vi "UHR-Fleezers Control (host) -TL FB Corrected Ronen semipassive - stepping.vi"(0 "Tab Control":T5(tab)=enum."Trap Control (RF)") -> ()   [LabVIEW 2013] (continued)
  n79 = xnode "Read/Write Control"("FPGA VI Reference In"=w138, "error in"=w158, "ai count"="AI Count (ticks)", "Interlace ON/OFF"=w124, "Number Interlace Cycles"=w123, "AI1 Sets to FIFO"=w251, "FB On/Off Set 1"=w250, "FB On/Off Set 2"=w249, "Interlace Off Parameters"=w122, "FB Setpoint Set 1"=w241, "FB Setpoint Set 2"=w240, "FB Gains Set 1"=w238, "FB Gains Set 2"=w237, "FB output range 1"=w140, "FB output range 2"=w140, "Cycles per step"=w222, "Scan BD"=w234, "Number of scans"=w218, "Scan steps"=w223, "Scan freq.  increment"=w224, "AO1"=w206, "AO2"=w205, "Scan freq.  increment (MCL)"=w199, "Scan steps (MCL)"=w198, "Cycles per step (MCL)"=w197, "Number of scans (MCL)"=w196, "MCL count"=w121, "Cont. Scan (MCL)"=w195, "MCL Scan Axis"=w189, "1D or 2D Scan?"=w141, "N of AI1 Int Acq Sets"=w179, "Freq or Amp switch first"="Freq or Amp switch first", "Freq switch delay"="Freq switch delay", "Amp switch delay"="Amp switch delay", "Swap F1 and F2"="Swap F1 and F2", "APD Acq Rate Count"=w146, "APD to FIFO"=FALSE, "APD Gate Operating Mode"="APD Gate", "APD Gate ON Count"="APD Gate ON Count", "APD Gate OFF Count"="APD Gate OFF Count", "Invert APD Gate"="Invert APD Gate", "DIO count 1 (ticks)"="DIO count 1 (ticks)", "DIO count 2 (ticks)"="DIO count 2 (ticks)", "DIO count 3 (ticks)"="DIO count 3 (ticks)", "APD 1 AO scale factor"="APD 1 AO Mult.", "APD 2 AO scale factor"="APD 2 AO Mult.", "Diff FB Measurement?"=w3, "Dynamic Force FB (Ronen)"=w2, "Negate Diff?"=w1) -> ("FPGA VI Reference Out"=w116:T20, "error out"=w118:errorcluster)  [unwired: 1 in]
  n80 = local read "Green Laser ON/Interlacing"() -> (w119:bool)
  n81 = local read "Green laser mode"() -> (w120:enum32{"Laser ON", "Laser OFF", "Interlace"})
  n82 = local read "GI Frequency, OFF count"() -> (w112:u32)
  n83 = local read "GI Frequency, ON count"() -> (w111:u32)
  n84 = Multiply(x="Current When FB OFF (%)", y=655.35) -> (x*y=w102:dbl)
  n85 = local read "Green FB Count"() -> (w110:u32)
  n86 = Multiply(x="Green FB Setpoint (mV)", y=3.2767) -> (x*y=w99:dbl)
  n87 = To Unsigned Word Integer(number=w102) -> (unsigned 16bit integer=w100:u16)
  n88 = local read "Invert GI"() -> (w114:bool)
  n89 = To Word Integer(number=w99) -> (16bit integer=w97:i16)
  n90 = case shown="True" w119 {
    tunnel: w120 -> [_ w271]
    tunnel: [enum32{"Laser ON", "Laser OFF", "Interlace"}."Laser OFF" ("Green laser mode") w271] -> w113
    frame False {
    }
    frame True {
    }
  }
  n91 = local read "Trap Pos. AI1 X Pre-scale"() -> (w68:u16)
  n92 = local read "Trap Pos FB Monitor\nT1 or T2"() -> (w75:bool)
  n93 = local read "Trap Pos FB Int Count"() -> (w63:u16)
  n94 = local read "Trap Pos FB Negate Action"() -> (w74:bool)
  n95 = local read "Trap Pos. FB Offset Factor"() -> (w73:i64)
  n96 = local read "Trap Pos. FB Mult Factor"() -> (w72:i64)
  n97 = local read "Trap Pos. FB Gains"() -> (w70:T11)
  n98 = local read "Trap Pos. FB Range"() -> (w71:T12)
  n99 = xnode "Read/Write Control"("FPGA VI Reference In"=w116, "error in"=w118, "Green interlace ON count 2"=w111, "Green interlace OFF count 2"=w112, "Invert GI 2"=w114, "Operating Mode 2"=w113, "Green FB Gains"="Green FB Gains", "Green FB Setpoint"=w97, "Green FB On/Off"="Green FB On/Off", "Current Out"=w100, "Green int current ON count adj"="Green int current ON count adj", "Green FB Count"=w110, "Operating Mode"=w113, "Green interlace OFF count"=w112, "Green interlace ON count"=w111, "Invert GI"=w114, "Trap Pos FB Monitor T1 or T2"=w75, "Trap Pos FB Negate Action"=w74, "Trap Pos. FB Offset Factor"=w73, "Trap Pos. FB Mult Factor"=w72, "Trap Pos. FB Range"=w71, "Trap Pos. FB Gains"=w70, "Force feedback"=FALSE, "AI1 X Scale"=w68, "Trap Pos to FIFO"=TRUE, "Trap Pos FB Int Count"=w63) -> ("FPGA VI Reference Out"=w115:T20, "error out"=w117:errorcluster)
  n100 = xnode "Invoke Method"("FPGA VI Reference In"=w115, "error in"=w117, "Requested Depth"="Trap AI FIFO Depth") -> ("FPGA VI Reference Out"=w78:T20, "error out"=w77:errorcluster)  [unwired: 1 out]
  n101 = xnode "Invoke Method"("FPGA VI Reference In"=w78, "error in"=w77, "Requested Depth"="Trap Position FIFO Depth") -> ("FPGA VI Reference Out"=w65:T20, "error out"=w64:errorcluster)  [unwired: 1 out]
  n102 = flat-sequence {
    tunnel: w139 -> [w276]
    tunnel: [w276] -> w138
    tunnel: [w275] -> w20
    tunnel: [w274] -> w137
    tunnel: [w272] -> w135
    tunnel: [w273] -> w136
    frame #0 {
      w273 = T17 {"Minimum"=60.0, "Maximum"=90.0, "Increment"=1.0} ("Min Max Inc")
      w272 = T17 {"Minimum"=0.0, "Maximum"=75.0, "Increment"=1.0} ("Data Entry Limits")
      w275 = T17 {"Minimum"=60.0, "Maximum"=90.0, "Increment"=1.0} ("Min Max Inc")
      w274 = T17 {"Minimum"=0.0, "Maximum"=75.0, "Increment"=1.0} ("Data Entry Limits")
      n103 = property on="BD 2 Frequency 1 (MHz)" class="DigNum (strict)"("Data Range"=w273) -> ()  [unwired: 2 in, 2 out]
      n104 = property on="BD 2 Frequency 3 (MHz)" class="DigNum (strict)"("Data Range"=w273) -> ()  [unwired: 2 in, 2 out]
      n105 = property on="BD 2 Frequency 2 (MHz)" class="DigNum (strict)"("Data Range"=w273) -> ()  [unwired: 2 in, 2 out]
      n106 = property on="BD 1 Frequency 1 (MHz)" class="DigNum (strict)"("Data Range"=w275) -> ()  [unwired: 2 in, 2 out]
      n107 = property on="BD 1 Frequency 2 (MHz)" class="DigNum (strict)"("Data Range"=w275) -> ()  [unwired: 2 in, 2 out]
      n108 = property on="BD 1 Frequency 3 (MHz)" class="DigNum (strict)"("Data Range"=w275) -> ()  [unwired: 2 in, 2 out]
      n109 = property on="BD 2 Amplitude 1 (%)" class="DigNum (strict)"("Data Range"=w272) -> ()  [unwired: 2 in, 2 out]
      n110 = property on="BD 2 Amplitude 2 (%)" class="DigNum (strict)"("Data Range"=w272) -> ()  [unwired: 2 in, 2 out]
      n111 = property on="BD 2 Amplitude 3 (%)" class="DigNum (strict)"("Data Range"=w272) -> ()  [unwired: 2 in, 2 out]
      n112 = property on="BD 1 Amplitude 3 (%)" class="DigNum (strict)"("Data Range"=w274) -> ()  [unwired: 2 in, 2 out]
      n113 = property on="BD 1 Amplitude 2 (%)" class="DigNum (strict)"("Data Range"=w274) -> ()  [unwired: 2 in, 2 out]
      n114 = property on="BD 1 Amplitude 1 (%)" class="DigNum (strict)"("Data Range"=w274) -> ()  [unwired: 2 in, 2 out]
      "X RF Frequency Limits (MHz)" <- w275
      "X RF Amplitude Limits (%)" <- w274
      "Y RF Amplitude Limits (%)" <- w272
      "Y RF Frequency Limits (MHz)" <- w273
    }
  }
  n115 = xnode "Invoke Method"("FPGA VI Reference In"=w65, "error in"=w64) -> ("FPGA VI Reference Out"=w42:T20, "error out"=w41:errorcluster)  [unwired: 1 in]
  n116 = flat-sequence "Initial FPGA Loop Relative Phase Adjustment" {
    tunnel: "Initial Phase Adjustment (APD 2 Gate)" -> [w278]
    tunnel: "Initial Phase Adjustment (GI) 2" -> [w279]
    tunnel: "Initial Phase Adj. (MCL)" -> [w280]
    tunnel: w41 -> [w281]
    tunnel: w42 -> [w282]
    tunnel: "Initial Phase Adjustment (GI)" -> [w283]
    tunnel: "Initial Phase Adjustment (AI1)" -> [w284]
    tunnel: [w284] -> w51
    tunnel: [w283] -> w50
    tunnel: [w282] -> w49
    tunnel: [w281] -> w48
    tunnel: [w280] -> w47
    tunnel: [w279] -> w46
    tunnel: [w278] -> w45
    tunnel: [w296] -> w164
    tunnel: [w290] -> w162
    tunnel: "Initial Phase Adjustment (APD Acq)" -> [w289]
    tunnel: "Initial Phase Adjustment (APD 1 Gate)" -> [w288]
    tunnel: "Initial Phase Adjustment (Green FB)" -> [w287]
    tunnel: w51 -> [w295]
    tunnel: w50 -> [w294]
    tunnel: w49 -> [w293]
    tunnel: w48 -> [w292]
    tunnel: w47 -> [w291]
    tunnel: w46 -> [w286]
    tunnel: w45 -> [w285]
    tunnel: w164 -> [w298]
    tunnel: [w299] -> w163
    tunnel: w162 -> [w299]
    tunnel: [w298] -> w161
    tunnel: w163 -> [w302]
    tunnel: w161 -> [w301]
    tunnel: [w304] -> w160
    tunnel: [w303] -> w159
    tunnel: [w306] -> w40
    tunnel: [w307] -> w43
    tunnel: w160 -> [w307]
    tunnel: w159 -> [w306]
    frame #0 {
      n117 = Wait (ms)(milliseconds to wait=u32 1000) -> ()  [unwired: 1 out]
    }
    frame #1 {
      n118 = xnode "Read/Write Control"("FPGA VI Reference In"=w293, "error in"=w292, "Phase count adjustment"=w295, "Phase count adjustment (GI)"=w294, "Phase count adjustment (MCL)"=w291, "Phase Count Adjustment (APD Acq)"=w289, "Phase count adjustment (APD 1 Gate)"=w288, "Phase count adjustment (APD 2 Gate)"=w285, "Phase count adjustment (Green FB)"=w287, "Phase count adjustment (GI) 2"=w286) -> ("FPGA VI Reference Out"=w290:T20, "error out"=w296:errorcluster)
    }
    frame #2 {
      n119 = Wait (ms)(milliseconds to wait=u32 1000) -> ()  [unwired: 1 out]
    }
    frame #3 {
      w300 = TRUE
      n120 = xnode "Read/Write Control"("FPGA VI Reference In"=w302, "error in"=w301, "+ phase"=w300, "+ phase (GI)"=w300, "+ phase (MCL)"=w300, "+ phase (APD Acq)"=w300, "+ phase (APD 1 Gate)"=w300, "+ phase (APD 2 Gate)"=w300, "+ phase (Green FB)"=w300, "+ phase (GI) 2"=w300) -> ("FPGA VI Reference Out"=w303:T20, "error out"=w304:errorcluster)
    }
    frame #4 {
      n121 = Wait (ms)(milliseconds to wait=u32 1000) -> ()  [unwired: 1 out]
    }
  }
  n122 = Unbundle By Name(w20) -> ("Minimum"=w19:dbl, "Maximum"=w18:dbl)
  n123 = local read "Phase adj. (Green FB)"() -> (w133:i16)
  n124 = local read "Phase adj. (GI) 2"() -> (w103:i16)
  n125 = local read "Phase adjust (MCL)"() -> (w190:i16)
  n126 = local read "Phase adj. (AI1)"() -> (w192:i16)
  n127 = local read "Phase adj. (GI)"() -> (w191:i16)
  n128 = Multiply(x=w19, y=w17) -> (x*y=w15:dbl)
  n129 = Multiply(x=w18, y=w17) -> (x*y=w16:dbl)
  n130 = Multiply(x=49152000.0, y=6.0) -> (x*y=w9:dbl)
  n131 = Scale By Power Of 2(n=w14, x=w15) -> (x*2^n=w11:dbl)
  n132 = Scale By Power Of 2(n=w14, x=w16) -> (x*2^n=w10:dbl)
  n133 = xnode "Read/Write Control"("FPGA VI Reference In"=w40, "error in"=w43, "Phase count adjustment"=w192, "Phase count adjustment (GI)"=w191, "Phase count adjustment (MCL)"=w190, "Phase Count Adjustment (APD Acq)"="Phase Adj. (APD Acq)", "Phase count adjustment (APD 1 Gate)"="Phase Adj. (APD 1 Gate)", "Phase count adjustment (APD 2 Gate)"="Phase Adj. (APD 2 Gate)", "Phase count adjustment (Green FB)"=w133, "Phase count adjustment (GI) 2"=w103) -> ("FPGA VI Reference Out"=w39:T20, "error out"=w38:errorcluster)
  n134 = Divide(x=w10, y=w9) -> (x/y=w7:dbl)
  n135 = Divide(x=w11, y=w9) -> (x/y=w8:dbl)
  n136 = To Unsigned Quad Integer(1:w8) -> (0:w5:u64)
  n137 = To Unsigned Quad Integer(1:w7) -> (0:w4:u64)
  n138 = call "Initialize RF boards - interlace 3.vi"("error in"=w38, "FPGA VI Reference In"=w39) -> ("FPGA VI Reference Out"=w6:T20)  [unwired: 1 out]
  n139 = xnode "Read/Write Control"("FPGA VI Reference In"=w6, "FB Min Frequency"=w5, "FB Max Frequency"=w4) -> ()  [unwired: 1 in, 2 out]
  n140 = call "set RF board frequency - interlace.vi"("Board 2 Frequency Limits"=w136, "Board 1 Frequency Limits"=w20, "FPGA VI Reference In"=w6, "Board 2 Frequency 3 (MHz)"="BD 2 Frequency 3 (MHz)", "Board 1 Frequency 3 (MHz)"="BD 1 Frequency 3 (MHz)", "Board 2 Frequency 2 (MHz)"="BD 2 Frequency 2 (MHz)", "Board 2 Frequency 1 (MHz)"="BD 2 Frequency 1 (MHz)", "Board 1 Frequency 2 (MHz)"="BD 1 Frequency 2 (MHz)", "Board 1 Frequency 1  (MHz)"="BD 1 Frequency 1 (MHz)") -> ("error out"=w262:errorcluster, "FPGA VI Reference Out"=w263:T20)  [unwired: 1 in]
  n141 = call "set RF board amplitude - interlace.vi"("Board 2 Amplitude Limits"=w135, "Board 1 Amplitude Limits"=w137, "error in"=w262, "FPGA VI Reference In"=w263, "Board 2 Amplitude 3 (%)"="BD 2 Amplitude 3 (%)", "Board 1 Amplitude 3 (%)"="BD 1 Amplitude 3 (%)", "Board 2 Amplitude 2 (%)"="BD 2 Amplitude 2 (%)", "Board 2 Amplitude 1 (%)"="BD 2 Amplitude 1 (%)", "Board 1 Amplitude 2 (%)"="BD 1 Amplitude 2 (%)", "Board 1 Amplitude 1 (%)"="BD 1 Amplitude 1 (%)") -> ("error out"=w36:errorcluster, "FPGA VI Reference Out"=w37:T20)
  n142 = flat-sequence {
    tunnel: w37 -> [w316]
    tunnel: w36 -> [w315]
    tunnel: [w314] -> w255
    tunnel: [w313] -> w254
    tunnel: [w320] -> w253
    tunnel: w255 -> [w320]
    tunnel: [w319] -> w252
    tunnel: w254 -> [w319]
    tunnel: w253 -> [w329]
    tunnel: w252 -> [w328]
    tunnel: [w327] -> w32
    tunnel: [w322] -> w31
    tunnel: [w332] -> w60
    tunnel: [w336] -> w44
    tunnel: w32 -> [w336]
    tunnel: w31 -> [w331]
    frame #0 {
      n143 = local read "Trap 1 (ON/OFF)"() -> (w308:bool)
      n144 = xnode "Read/Write Control"("FPGA VI Reference In"=w316, "error in"=w315, "Direct RF Box  Communication"=FALSE) -> ("FPGA VI Reference Out"=w314:T20, "error out"=w313:errorcluster)
      n145 = local write "Saving..."(FALSE ("Saving Data")) -> ()
      n146 = local write "Stop All"(FALSE ("Stop All")) -> ()
      n147 = local write "Index"(1.0 ("Index")) -> ()
      n148 = property on="Trap 1 ON" class="Bool (strict)"("Value"=w308) -> ()  [unwired: 2 in, 2 out]
      "Manipulating Trap" <- FALSE ("Manipulating Trap")
    }
    frame #1 {
      n149 = local read "Trap 2 (ON/OFF)"() -> (w318:bool)
      n150 = Wait (ms)(milliseconds to wait=u32 50) -> ()  [unwired: 1 out]
      n151 = property on="Trap 2 ON" class="Bool (strict)"("Val(Sgnl)"=w318) -> ()  [unwired: 2 in, 2 out]
    }
    frame #2 {
      n152 = local read "Scan Range (nm)"() -> (w323:dbl)
      n153 = xnode "Read/Write Control"("FPGA VI Reference In"=w329, "error in"=w328, "FPGA Controls  RF Box"=TRUE ("Direct RF Box  Communication")) -> ("FPGA VI Reference Out"=w327:T20, "error out"=w322:errorcluster)
      n154 = call "Update messages.vi"("Message to add"="UHR-Fleezers ready.", "Old message string"="") -> ("New message string"=w326:string)
      n155 = local write "Messages"(w326) -> ()
      n156 = property on="Scan Range (nm)" class="DigNum (strict)"("Val(Sgnl)"=w323) -> ()  [unwired: 2 in, 2 out]
    }
    frame #3 {
      n157 = call "hamilton_controller.vi"("error in"=w331, "action"=T21."CONNECT") -> ("error out"=w333:errorcluster)  [unwired: 9 in]
      n158 = call "hamilton_controller.vi"("error in"=w333, "action"=T21."INITIALIZE VALVES") -> ("error out"=w332:errorcluster)  [unwired: 9 in]
    }
  }
  n159 = Subtract(x="BD 1 Frequency 1 (MHz)", y="BD 1 Frequency 2 (MHz)") -> (x-y=w178:dbl)
  n160 = Subtract(x="BD 2 Frequency 1 (MHz)", y="BD 2 Frequency 2 (MHz)") -> (x-y=w177:dbl)
  n161 = Square(x=w177) -> (x^2=w175:dbl)
  n162 = Square(x=w178) -> (x^2=w176:dbl)
  n163 = Add(x=w176, y=w175) -> (x+y=w174:dbl)
  n164 = Square Root(x=w174) -> (sqrt(x)=w173:dbl)
  n165 = local write "Trap Delta (MHz)"(w173) -> ()
  n166 = call "IMAQ Create"("Image Name"="APD 1 Image", "Image Type"=w84) -> ("New Image"=w83:T3)  [unwired: 3 in, 1 out]
  n167 = call "IMAQ Create"("Image Name"="APD 2 Image", "Image Type"=w84) -> ("New Image"=w82:T3)  [unwired: 3 in, 1 out]
  n168 = call "IMAQ Create"("Image Name"="Det. X Image", "Image Type"=w84) -> ("New Image"=w81:T3)  [unwired: 3 in, 1 out]
  n169 = call "IMAQ Create"("Image Name"="Det. Y Image", "Image Type"=w84) -> ("New Image"=w80:T3)  [unwired: 3 in, 1 out]
  n170 = Bundle("New Image"=w83, "New Image"=w82, "New Image"=w81, "New Image"=w80) -> (w79:T22)  [unwired: 1 in]
  n171 = Current VI's Path() -> (path=w21:path)
  n172 = Concatenate Strings("N.D.", "\r\n") -> (w25:string)
  n173 = Strip Path(path=w21) -> (stripped path=w22:path)  [unwired: 1 out]
  n174 = Initialize Array(w25, 4, 3) -> (w28:string[][])
  n175 = Build Path(base path=w22, name or relative path="Locations.txt") -> (appended path=→"Location path":path)
  n176 = local write "Location Matrix"(w28) -> ()
  n177 = while {
    stop <- w337 stop-if-true
    n178 = event shown="[0] Timeout" {
      selector: _ -> [_ _ _ _ _ _ _ _]
      dyn-events: _ -> [_ _ _ _ _ _ _ _]
      timeout: 10 -> [_ _ _ _ _ _ _ _]
      tunnel: [FALSE _ _ _ _ _ _ TRUE] -> w337
      event Timeout {
        # "Change the trajectory mode to Jog"
        # "Query and display stage positions"
        # "Setting ESP300 left and right limits for Z-axis, input in mm"
        # "Display Selected Location"
        n179 = event-data() -> ()  [unwired: 1 in, 2 out]
        n180 = local read "Capture Locations"() -> (w362:i32)
        n181 = local read "Location Matrix"() -> (w363:string[][])
        n182 = Concatenate Strings("1TP;\n2TP;\n3TP;\n1MD?;\n2MD?;\n3MD?" ("Substring"), "\r") -> (w346:string)
        n183 = local read "ESP Port"() -> (w349:refnum<visa-resource-name>)
        n184 = Index Array(array=w363, index (row)=w362) -> (element=w361:string[])  [unwired: 1 in]
        n185 = local read "ESP Port"() -> (w358:refnum<visa-resource-name>)
        n186 = VISA Write(VISA resource name=w349, write buffer=w346, error in (no error)="error in") -> (VISA resource name out=w347:refnum<visa-resource-name>, error out=w345:errorcluster)  [unwired: 1 out]
        n187 = Concatenate Strings("3SL" ("Substring"), "ESP ZL-Limit", ";3SR", "ESP ZR-Limit", "\r") -> (w357:string)
        n188 = Array To Cluster(array=w361) -> (cluster=w360:T23)
        n189 = case shown="True" TRUE ("Case Constant\n(See Context Help)") {
          tunnel: w347 -> [_ w401]
          tunnel: w345 -> [w382 w400]
          tunnel: [w382 w384] -> w351
          frame False {
          }
          frame True {
            w394 = u16 10 items=["1.0"=10, "1.5"=15, "2.0"=20] ("Serial Settings:Stop Bits")
            w395 = u16 0 items=["None", "Odd", "Even", "Mark", "Space"] ("Serial Settings:Parity")
            n190 = property class="Instr"(reference=w401, error in=w400, "Baud"=u32 921600 ("Serial Settings:Baud Rate"), "Data Bits"=u16 8 ("Serial Settings:Data Bits"), "Parity"=w395, "Stop Bits"=w394) -> (reference out=w399:refnum<visa-resource-name>, error out=w398:errorcluster, "Bytes at Port"=w383:u32)
            n191 = Wait (ms)(milliseconds to wait=u32 10) -> ()  [unwired: 1 out]
            n192 = VISA Read(VISA resource name=w399, byte count=w383, error in (no error)=w398) -> (VISA resource name out=w407:refnum<visa-resource-name>, read buffer=→"X Pos":string, error out=w408:errorcluster)  [unwired: 1 out]
            n193 = VISA Read(VISA resource name=w407, byte count=w383, error in (no error)=w408) -> (VISA resource name out=w405:refnum<visa-resource-name>, read buffer=→"Y Pos":string, error out=w406:errorcluster)  [unwired: 1 out]
            n194 = VISA Read(VISA resource name=w405, byte count=w383, error in (no error)=w406) -> (VISA resource name out=w393:refnum<visa-resource-name>, read buffer=→"Z Pos Pos":string, error out=w392:errorcluster)  [unwired: 1 out]
            n195 = VISA Read(VISA resource name=w393, byte count=w383, error in (no error)=w392) -> (VISA resource name out=w389:refnum<visa-resource-name>, read buffer=→"X Motion":string, error out=w390:errorcluster)  [unwired: 1 out]
            n196 = VISA Read(VISA resource name=w389, byte count=w383, error in (no error)=w390) -> (VISA resource name out=w388:refnum<visa-resource-name>, read buffer=→"Y Motion":string, error out=w386:errorcluster)  [unwired: 1 out]
            n197 = VISA Read(VISA resource name=w388, byte count=w383, error in (no error)=w386) -> (read buffer=→"Z motion":string, error out=w384:errorcluster)  [unwired: 2 out]
          }
        }
        "error out" <- w351
        n198 = VISA Write(VISA resource name=w358, write buffer=w357) -> ()  [unwired: 1 in, 3 out]
        n199 = local write item#485(w360) -> ()
        n200 = disable-structure shown="Disabled" {
          frame Disabled {
            # "Change Low Jog Velocity"
            # "Change High Jog Velocity"
            n201 = Concatenate Strings("1JH" ("Substring"), "Axis 1", "2JH" ("Substring"), "Axis 2", "3JH" ("Substring"), "Axis 3", "\r") -> (w381:string)
            n202 = local read "ESP Port"() -> (w380:refnum<visa-resource-name>)
            n203 = VISA Write(VISA resource name=w380, write buffer=w381) -> ()  [unwired: 1 in, 3 out]
            n204 = Concatenate Strings("1JW" ("Substring"), "Axis 1", "2JW" ("Substring"), "Axis 2", "3JW" ("Substring"), "Axis 3", "\r") -> (w372:string)
            n205 = local read "ESP Port"() -> (w371:refnum<visa-resource-name>)
            n206 = VISA Write(VISA resource name=w371, write buffer=w372) -> ()  [unwired: 1 in, 3 out]
          }
          frame Enabled {
          }
        }
        n207 = local read "ESP Port"() -> (w339:refnum<visa-resource-name>)
        n208 = Concatenate Strings("1TJ3;\n2TJ3;\n3TJ3" ("Substring"), "\r") -> (w340:string)
        n209 = VISA Write(VISA resource name=w339, write buffer=w340) -> ()  [unwired: 1 in, 3 out]
      }
      event "Goto Top (F6)": Value Change {
        n210 = event-data() -> ()  [unwired: 1 in, 5 out]
        n211 = stacked-sequence {
          frame #0 {
            # "stop motions of all axes before going to avoid reversing of direction"
            n212 = local read "ESP Port"() -> (w413:refnum<visa-resource-name>)
            n213 = Concatenate Strings("ST" ("Substring"), "\r") -> (w410:string)
            n214 = VISA Write(VISA resource name=w413, write buffer=w410) -> ()  [unwired: 1 in, 3 out]
          }
          frame #1 {
            n215 = Wait (ms)(milliseconds to wait=u32 50) -> ()  [unwired: 1 out]
          }
          frame #2 {
            # "Change the trajectory mode to Trapezoidal"
            n216 = local read "ESP Port"() -> (w418:refnum<visa-resource-name>)
            n217 = Concatenate Strings("1TJ1;\n2TJ1;\n3TJ1" ("Substring"), "\r") -> (w415:string)
            n218 = VISA Write(VISA resource name=w418, write buffer=w415) -> ()  [unwired: 1 in, 3 out]
          }
          frame #3 {
            # "Go to Top Dispensor"
            n219 = local read "Location Matrix"() -> (w430:string[][])
            n220 = Index Array(array=w430, index (row)=0) -> (element=w426:string[])  [unwired: 1 in]
            n221 = Decimate 1D Array(w426) -> (w424:string[], w422:string[], w420:string[])
            n222 = local read "ESP Port"() -> (w427:refnum<visa-resource-name>)
            n223 = Concatenate Strings("1PA" ("Substring"), w424, "2PA" ("Substring"), w422, "3PA" ("Substring"), w420, "\r") -> (w428:string)
            n224 = VISA Write(VISA resource name=w427, write buffer=w428) -> ()  [unwired: 1 in, 3 out]
          }
          frame #4 {
            n225 = Wait (ms)(milliseconds to wait=u32 100) -> ()  [unwired: 1 out]
          }
          frame #5 {
            # "Change the trajectory mode to Jog"
            n226 = local read "ESP Port"() -> (w435:refnum<visa-resource-name>)
            n227 = Concatenate Strings("1TJ3;\n2TJ3;\n3TJ3" ("Substring"), "\r") -> (w432:string)
            n228 = VISA Write(VISA resource name=w435, write buffer=w432) -> ()  [unwired: 1 in, 3 out]
          }
        }
      }
      event "Goto Exp (F8)": Value Change {
        n229 = event-data() -> ()  [unwired: 1 in, 5 out]
        n230 = stacked-sequence {
          frame #0 {
            # "stop motions of all axes before going to avoid reversing of direction"
            n231 = local read "ESP Port"() -> (w439:refnum<visa-resource-name>)
            n232 = Concatenate Strings("ST" ("Substring"), "\r") -> (w436:string)
            n233 = VISA Write(VISA resource name=w439, write buffer=w436) -> ()  [unwired: 1 in, 3 out]
          }
          frame #1 {
            n234 = Wait (ms)(milliseconds to wait=u32 50) -> ()  [unwired: 1 out]
          }
          frame #2 {
            # "Change the trajectory mode to Trapezoidal"
            n235 = local read "ESP Port"() -> (w444:refnum<visa-resource-name>)
            n236 = Concatenate Strings("1TJ1;\n2TJ1;\n3TJ1" ("Substring"), "\r") -> (w441:string)
            n237 = VISA Write(VISA resource name=w444, write buffer=w441) -> ()  [unwired: 1 in, 3 out]
          }
          frame #3 {
            # "Go to Experimental"
            n238 = local read "Location Matrix"() -> (w456:string[][])
            n239 = Index Array(array=w456, index (row)=2) -> (element=w452:string[])  [unwired: 1 in]
            n240 = Decimate 1D Array(w452) -> (w450:string[], w448:string[], w446:string[])
            n241 = Concatenate Strings("1PA" ("Substring"), w450, "2PA" ("Substring"), w448, "3PA" ("Substring"), w446, "\r") -> (w454:string)
            n242 = local read "ESP Port"() -> (w453:refnum<visa-resource-name>)
            n243 = VISA Write(VISA resource name=w453, write buffer=w454) -> ()  [unwired: 1 in, 3 out]
          }
          frame #4 {
            n244 = Wait (ms)(milliseconds to wait=u32 200) -> ()  [unwired: 1 out]
          }
          frame #5 {
            # "Change the trajectory mode to Jog"
            n245 = local read "ESP Port"() -> (w458:refnum<visa-resource-name>)
            n246 = Concatenate Strings("1TJ3;\n2TJ3;\n3TJ3" ("Substring"), "\r") -> (w461:string)
            n247 = VISA Write(VISA resource name=w458, write buffer=w461) -> ()  [unwired: 1 in, 3 out]
          }
        }
      }
      event "Goto Bottom (F7)": Value Change {
        n248 = event-data() -> ()  [unwired: 1 in, 5 out]
        n249 = stacked-sequence {
          frame #0 {
            # "stop motions of all axes before going to avoid reversing of direction"
            n250 = local read "ESP Port"() -> (w465:refnum<visa-resource-name>)
            n251 = Concatenate Strings("ST" ("Substring"), "\r") -> (w462:string)
            n252 = VISA Write(VISA resource name=w465, write buffer=w462) -> ()  [unwired: 1 in, 3 out]
          }
          frame #1 {
            n253 = Wait (ms)(milliseconds to wait=u32 50) -> ()  [unwired: 1 out]
          }
          frame #2 {
            # "Change the trajectory mode to Trapezoidal"
            n254 = local read "ESP Port"() -> (w470:refnum<visa-resource-name>)
            n255 = Concatenate Strings("1TJ1;\n2TJ1;\n3TJ1" ("Substring"), "\r") -> (w467:string)
            n256 = VISA Write(VISA resource name=w470, write buffer=w467) -> ()  [unwired: 1 in, 3 out]
          }
          frame #3 {
            # "Go to Bottom Dispensor"
            n257 = local read "Location Matrix"() -> (w482:string[][])
            n258 = Index Array(array=w482, index (row)=1) -> (element=w478:string[])  [unwired: 1 in]
            n259 = Decimate 1D Array(w478) -> (w476:string[], w474:string[], w472:string[])
            n260 = Concatenate Strings("1PA" ("Substring"), w476, "2PA" ("Substring"), w474, "3PA" ("Substring"), w472, "\r") -> (w480:string)
            n261 = local read "ESP Port"() -> (w479:refnum<visa-resource-name>)
            n262 = VISA Write(VISA resource name=w479, write buffer=w480) -> ()  [unwired: 1 in, 3 out]
          }
          frame #4 {
            n263 = Wait (ms)(milliseconds to wait=u32 200) -> ()  [unwired: 1 out]
          }
          frame #5 {
            # "Change the trajectory mode to Jog"
            n264 = local read "ESP Port"() -> (w484:refnum<visa-resource-name>)
            n265 = Concatenate Strings("1TJ3;\n2TJ3;\n3TJ3" ("Substring"), "\r") -> (w487:string)
            n266 = VISA Write(VISA resource name=w484, write buffer=w487) -> ()  [unwired: 1 in, 3 out]
          }
        }
      }
      event "Capture": Value Change {
        n267 = event-data() -> ()  [unwired: 1 in, 5 out]
        n268 = local read "Capture Locations"() -> (w488:i32)
        n269 = local read "Z Pos Pos"() -> (w489:string)
        n270 = local read "X Pos"() -> (w491:string)
        n271 = local read "Y Pos"() -> (w490:string)
        n272 = case shown="1" w488 {
          selector: w488 -> [w495 w502 w509 w516]
          tunnel: w491 -> [w498 w505 w512 w519]
          tunnel: w490 -> [w497 w504 w511 w518]
          tunnel: w489 -> [w496 w503 w510 w517]
          frame 0, Default {
            # "Capture Top Dispensor Location"
            n273 = local read "Location Matrix"() -> (w494:string[][])
            n274 = Build Array(w498, w497, w496) -> (w493:string[])
            n275 = Replace Array Subset(array=w494, new element=w493, index (row)=w495) -> (w492:string[][])  [unwired: 1 in]
            n276 = local write "Location Matrix"(w492) -> ()
          }
          frame 1 {
            # "Capture Bottom Dispensor Location"
            n277 = local read "Location Matrix"() -> (w501:string[][])
            n278 = Build Array(w505, w504, w503) -> (w500:string[])
            n279 = Replace Array Subset(array=w501, new element=w500, index (row)=w502) -> (w499:string[][])  [unwired: 1 in]
            n280 = local write "Location Matrix"(w499) -> ()
          }
          frame 2 {
            # "Capture Experimental Region Location"
            n281 = local read "Location Matrix"() -> (w508:string[][])
            n282 = Build Array(w512, w511, w510) -> (w507:string[])
            n283 = Replace Array Subset(array=w508, new element=w507, index (row)=w509) -> (w506:string[][])  [unwired: 1 in]
            n284 = local write "Location Matrix"(w506) -> ()
          }
          frame 3 {
            # "Capture Other Location"
            n285 = local read "Location Matrix"() -> (w515:string[][])
            n286 = Build Array(w519, w518, w517) -> (w514:string[])
            n287 = Replace Array Subset(array=w515, new element=w514, index (row)=w516) -> (w513:string[][])  [unwired: 1 in]
            n288 = local write "Location Matrix"(w513) -> ()
          }
        }
      }
      event "Save": Value Change {
        # "reshape Location Matrix to 1-D array to write"
        n289 = event-data() -> ()  [unwired: 1 in, 5 out]
        n290 = local read "Location Matrix"() -> (w523:string[][])
        n291 = local read "Location path"() -> (w520:path)
        n292 = Reshape Array(w523, 12) -> (w521:string[])
        n293 = Write to Text File(file (use dialog)=w520, text=w521) -> ()  [unwired: 2 in, 3 out]
      }
      event "Activate Joystick": Value Change {
        # "Change the trajectory mode to Jog"
        n294 = event-data() -> ()  [unwired: 1 in, 5 out]
        n295 = disable-structure shown="Disabled" {
          frame Disabled {
            n296 = case shown="True" "Activate Joystick" {
              frame False {
              }
              frame True {
                # "Change the trajectory mode to Jog"
                n297 = local read "ESP Port"() -> (w532:refnum<visa-resource-name>)
                n298 = Concatenate Strings("1TJ3;\n2TJ3;\n3TJ3" ("Substring"), "\r") -> (w529:string)
                n299 = VISA Write(VISA resource name=w532, write buffer=w529) -> ()  [unwired: 1 in, 3 out]
              }
            }
          }
          frame Enabled {
          }
        }
        n300 = local read "ESP Port"() -> (w524:refnum<visa-resource-name>)
        n301 = Concatenate Strings("1TJ3;\n2TJ3;\n3TJ3" ("Substring"), "\r") -> (w527:string)
        n302 = VISA Write(VISA resource name=w524, write buffer=w527) -> ()  [unwired: 1 in, 3 out]
      }
      event "Stop All": Mouse Down {
        n303 = event-data() -> ()  [unwired: 1 in, 5 out]
      }
    }
  }
  n304 = disable-structure shown="Disabled" {
    disable-tunnel: w44 -> [w562 _]
    frame Disabled {
      w557 = T18 0 items=["Grayscale (U8)", "Grayscale (I16)", "Grayscale (SGL)", "Complex (CSG)", "RGB (U32)", "HSL (U32)", "RGB (U64)", "Grayscale (U16)"] ("Image Type")
      n305 = call <vilib>:"IMAQ Init.vi"("Interface Name"="img0") -> ("error out"=w559:errorcluster, "IMAQ Session Out"=w561:refnum<k11>)  [unwired: 9 in]
      n306 = call <vilib>:"IMAQ Grab Setup.vi"("error in (no error)"=w559, "IMAQ Session In"=w561) -> ("error out"=w555:errorcluster, "IMAQ Session Out"=w556:refnum<k11>)  [unwired: 8 in]
      n307 = call "IMAQ Create"("Image Name"="untitled", "Image Type"=w557) -> ("New Image"=w554:T3)  [unwired: 3 in, 1 out]
      n308 = call <vilib>:"Application Directory.vi"() -> ("Application Directory"=w541:path)
      n309 = Build Path(base path=w541, name or relative path="_trap_screen_positions") -> (appended path=w549:path)
      n310 = Open/Create/Replace File(file path (use dialog)=w549, operation (0:open)=T24."open or create", access (0:read/write)=enum16{"read/write", "read-only", "write-only"}."read/write") -> (refnum out=w551:refnum<file>)  [unwired: 3 in, 2 out]
      n311 = local read "Trap Sets"() -> (w543:u32)
      n312 = for "Load trap positions on video screen from file." {
        N: w543 -> [_]
        tunnel: [w569] -> w544
        tunnel: w551 -> [w568]
        tunnel: [w565] -> w540 mode=indexing
        w567 = 4
        n313 = for {
          N: w567 -> [_]
          tunnel: [w573] -> w569
          tunnel: w568 -> [w572]
          tunnel: w567 -> [w571]
          tunnel: [w570] -> w566 mode=indexing
          n314 = Read from Binary File(5:w571, 11:w572) -> (2:w570:i32, 3:w573:refnum<file>)  [unwired: 4 in, 2 out]
        }
        n315 = Array To Cluster(array=w566) -> (cluster=w565:T28)
      }
      n316 = node-c288() -> (w564:T25)  [unwired: 4 in]
      n317 = timed-loop "acquire video and stage position" {
        timing: w564 -> [_]
        timing-out: [_] -> w563
        tunnel: w556 -> [w592]
        tunnel: w555 -> [w591]
        tunnel: w554 -> [w590]
        tunnel: [w589] -> w536
        tunnel: [w586] -> w537
        tunnel: [w587] -> w535
        tunnel: w562 -> [_]
        shift-right: [w583] -> w553
        shift-left: w540 -> [w584]
        tunnel: w543 -> [w581]
        stop <- w588 stop-if-true
        n318 = node-c288() -> ()  [unwired: 1 in, 1 out]
        n319 = event shown="[0] Timeout" {
          selector: _ -> [_ _ _ _]
          dyn-events: _ -> [_ _ _ _]
          timeout: 10 -> [_ _ _ _]
          tunnel: w592 -> [w603 w618 w627 w646]
          tunnel: w591 -> [w602 w620 w625 w648]
          tunnel: w590 -> [w601 w619 w626 w647]
          tunnel: [w600 w618 w627 w646] -> w589
          tunnel: [w593 w622 FALSE FALSE] -> w588
          tunnel: [w597 w620 w625 w648] -> w587
          tunnel: [w596 w619 w626 w647] -> w586
          tunnel: "radius" -> [_ _ w632 _]
          tunnel: w584 -> [w594 w621 w630 _]
          tunnel: [w594 w621 w631 cluster{i32, i32, i32, i32}[] []] -> w583
          tunnel: w581 -> [_ _ w623 _]
          event Timeout {
            n320 = event-data() -> ()  [unwired: 1 in, 2 out]
            n321 = call <vilib>:"IMAQ Grab Acquire.vi"("error in (no error)"=w602, "Image In"=w601, "IMAQ Session In"=w603) -> ("error out"=w598:errorcluster, "Image Out"=w599:T3, "IMAQ Session Out"=w600:refnum<k11>)  [unwired: 5 in, 1 out]
            n322 = case shown="True" "trap\nmarkers?" {
              tunnel: w594 -> [_ w611]
              tunnel: w599 -> [w605 w610]
              tunnel: w598 -> [w604 w609]
              tunnel: [w604 w608] -> w597
              tunnel: [w605 w606] -> w596
              frame False {
              }
              frame True {
                n323 = for {
                  tunnel: w611 -> [w617] mode=indexing
                  shift-right: [w615] -> w606
                  shift-left: w610 -> [w616]
                  tunnel: w609 -> [w614]
                  tunnel: [w613] -> w608
                  tunnel: u32 16711680 ("Color") -> [w612]
                  n324 = call "IMAQ Overlay Oval"("Color"=w612, "error in (no error)"=w614, "Bounding Rectangle"=w617, "Image"=w616) -> ("error out"=w613:errorcluster, "Image Out"=w615:T3)  [unwired: 6 in]
                }
              }
            }
            "Primary Video Display" <- w596
            n325 = Unbundle By Name(w598) -> ("status"=w593:bool)
          }
          event "Stop All": Value Change {
            n326 = event-data() -> ()  [unwired: 1 in, 5 out]
            n327 = local read "Stop All"() -> (w622:bool)
          }
          event "Primary Video Display": Mouse Down {
            n328 = event-data() -> ()  [unwired: 1 in, 7 out]
            n329 = Array Size(array=w630) -> (size(s)=w629:i32)
            n330 = Less?(x=w629, y=w623) -> (x < y?=w628:bool)
            n331 = case shown="True" w628 {
              tunnel: w632 -> [_ w642]
              tunnel: w630 -> [w633 w636]
              tunnel: [w633 w635] -> w631
              frame False {
              }
              frame True {
                n332 = property on="Primary Video Display" class="ImageControl"() -> ("Last Mouse Position"=w634:cluster{"X":i32, "Y":i32})  [unwired: 2 in, 2 out]
                n333 = Unbundle By Name(w634) -> ("X"=w644:i32, "Y"=w643:i32)
                n334 = Add(x=w643, y=w642) -> (x+y=w640:i32)
                n335 = Subtract(x=w643, y=w642) -> (x-y=w638:i32)
                n336 = Add(x=w644, y=w642) -> (x+y=w639:i32)
                n337 = Subtract(x=w644, y=w642) -> (x-y=w641:i32)
                n338 = Bundle(w641, w640, w639, w638) -> (w637:cluster{i32, i32, i32, i32})  [unwired: 1 in]
                n339 = Build Array (concatenate)(w636, w637) -> (w635:T29)
              }
            }
          }
          event "clear markers": Value Change {
            n340 = event-data() -> ()  [unwired: 1 in, 5 out]
          }
        }
        n341 = node-c288() -> ()  [unwired: 1 in, 1 out]
      }
      n342 = node-c288(w563) -> ()  [unwired: 1 out]
      n343 = Set File Position(offset (in bytes) (0)=i64 0, refnum=w544, from (0:start)=enum16{"start", "end", "current"}."start") -> (refnum out=w545:refnum<file>)  [unwired: 1 in, 1 out]
      n344 = for "Write trap positions to file so they can be remembered\nwhen program is removed from memory" {
        tunnel: w553 -> [w577] mode=indexing
        tunnel: [w575] -> w552
        tunnel: w545 -> [w574]
        n345 = Cluster To Array(cluster=w577) -> (array=w576:i32[])
        n346 = for {
          tunnel: w576 -> [w580] mode=indexing
          tunnel: [w579] -> w575
          tunnel: w574 -> [w578]
          n347 = Write to Binary File(file (use dialog)=w578, data=w580) -> (refnum out=w579:refnum<file>)  [unwired: 4 in, 2 out]
        }
      }
      n348 = Close File(refnum=w552) -> ()  [unwired: 1 in, 2 out]
      n349 = call "IMAQ Dispose"("Image"=w537, "error in (no error)"=w535) -> ("error out"=w534:errorcluster)  [unwired: 4 in]
      n350 = call <vilib>:"IMAQ Stop.vi"("error in (no error)"=w534, "IMAQ Session In"=w536) -> ("error out"=w538:errorcluster, "IMAQ Session Out"=w539:refnum<k11>)  [unwired: 8 in]
      n351 = call <vilib>:"IMAQ Close.vi"("error in (no error)"=w538, "IMAQ Session In"=w539) -> ()  [unwired: 9 in, 1 out]
    }
    frame Enabled {
    }
  }
  n352 = disable-structure shown="Enabled" {
    disable-tunnel: [w655 _] -> w55
    disable-tunnel: w44 -> [w654 _]
    frame Enabled {
      n353 = node-c288() -> (w657:T25)  [unwired: 4 out]
      n354 = timed-loop "Rough control of MCL mirror stage (debugging)" {
        tunnel: w654 -> [w660]
        tunnel: [w659] -> w655
        timing: w657 -> [_]
        timing-out: [_] -> w656
        stop <- w659 stop-if-true
        n355 = node-c288() -> ()  [unwired: 2 out]
        n356 = case shown="1" "MCL Mode" {
          tunnel: w660 -> [_ w663 w710]
          frame 0, Default {
            # "manual positioning"
          }
          frame 1 {
            # "sinusoidal wave"
            n357 = node-c288() -> (w665:T25)  [unwired: 4 out]
            n358 = timed-loop "Oscillate MCL mirror" {
              timing: w665 -> [_]
              timing-out: [_] -> w664
              tunnel: w663 -> [w704]
              i -> [w703]
              stop <- w666 stop-if-true
              n359 = node-c288() -> (w702:i64)  [unwired: 1 out]
              n360 = Multiply(x="AO1", y=32767.0) -> (x*y=w698:dbl)
              n361 = Multiply(x="AO2", y=32767.0) -> (x*y=w693:dbl)
              n362 = Divide(x=w698, y=10.0) -> (x/y=w699:dbl)
              n363 = Divide(x=w693, y=10.0) -> (x/y=w694:dbl)
              n364 = To Word Integer(number=w699) -> (16bit integer=w691:i16)
              n365 = To Word Integer(number=w694) -> (16bit integer=w690:i16)
              n366 = Divide(x=w702, y=i64 1000) -> (x/y=w673:dbl)
              n367 = Multiply(x=w673, y=w703) -> (x*y=w684:dbl)
              n368 = Multiply(x="Osc. freq. (Hz) 2", y=6.283185307179586) -> (x*y=w685:dbl)
              n369 = Multiply(x=w685, y=w684) -> (x*y=w683:dbl)
              n370 = Sine(x=w683) -> (sin(x)=w682:dbl)
              n371 = Multiply(x=w682, y="Osc. amp. (V)") -> (x*y=w680:dbl)
              n372 = Add(x=w680, y="Osc. center (V)") -> (x+y=w678:dbl)
              n373 = Divide(x=w678, y=10.0) -> (x/y=w676:dbl)
              n374 = Multiply(x=w676, y=32767.0) -> (x*y=w671:dbl)
              n375 = Select(t=w671, s="Scan axis", f=w691) -> (s? t:f=w689:dbl)
              n376 = Select(t=w690, s="Scan axis", f=w671) -> (s? t:f=w688:dbl)
              n377 = local read "MCL Mode"() -> (w670:u16)
              n378 = Not Equal?(x=w670, y=u16 1) -> (x != y?=w667:bool)
              n379 = local read "Stop All"() -> (w668:bool)
              n380 = xnode "Read/Write Control"("FPGA VI Reference In"=w704, "AO1"=w689, "AO2"=w688) -> ()  [unwired: 1 in, 2 out]
              n381 = Compound Arithmetic op=OR(w668, w667) -> (w666:bool)
              n382 = node-c288() -> ()  [unwired: 2 out]
            }
            n383 = node-c288(w664) -> ()  [unwired: 1 out]
          }
          frame 2 {
            # "linear scan"
            n384 = case shown="True" "Start Scan" {
              tunnel: w710 -> [_ w722]
              frame False {
              }
              frame True {
                n385 = Subtract(x="End (V)", y="Begin (V)") -> (x-y=w718:dbl)
                n386 = Decrement(x="N Points") -> (x-1=w717:dbl)
                n387 = Divide(x=w718, y=w717) -> (x/y=w715:dbl)
                n388 = for {
                  N: "N Points" -> [_]
                  tunnel: "Begin (V)" -> [w735]
                  tunnel: w722 -> [w727]
                  tunnel: [w726] -> w721 mode=indexing
                  tunnel: w715 -> [w725]
                  tunnel: [w723] -> w714 mode=indexing
                  i -> [w734]
                  n389 = Multiply(x=w725, y=w734) -> (x*y=w733:dbl)
                  n390 = Add(x=w735, y=w733) -> (x+y=w730:dbl)
                  n391 = local read "Scan axis"() -> (w724:bool)
                  n392 = local read "AO1"() -> (w732:dbl)
                  n393 = local read "AO2"() -> (w731:dbl)
                  n394 = Select(t=w730, s=w724, f=w732) -> (s? t:f=w729:dbl)
                  n395 = Select(t=w731, s=w724, f=w730) -> (s? t:f=w728:dbl)
                  n396 = flat-sequence {
                    tunnel: w729 -> [w739]
                    tunnel: w728 -> [w738]
                    tunnel: w727 -> [w736]
                    tunnel: [w749] -> w726
                    tunnel: [w748] -> w723
                    frame #0 {
                      w742 = 10.0 ("y")
                      w737 = 32767.0 ("y")
                      n397 = Multiply(x=w739, y=w737) -> (x*y=w745:dbl)
                      n398 = Multiply(x=w738, y=w737) -> (x*y=w743:dbl)
                      n399 = Divide(x=w745, y=w742) -> (x/y=w746:dbl)
                      n400 = Divide(x=w743, y=w742) -> (x/y=w744:dbl)
                      n401 = To Word Integer(number=w746) -> (16bit integer=w740:i16)
                      n402 = To Word Integer(number=w744) -> (16bit integer=w741:i16)
                      n403 = xnode "Read/Write Control"("FPGA VI Reference In"=w736, "AO1"=w740, "AO2"=w741) -> ()  [unwired: 1 in, 2 out]
                    }
                    frame #1 {
                      n404 = Wait (ms)(milliseconds to wait="DAQ Delay (ms)") -> ()  [unwired: 1 out]
                    }
                    frame #2 {
                      n405 = local read "Slow mean"() -> (w749:dbl)
                      n406 = local read "Sigma"() -> (w748:dbl)
                    }
                  }
                }
                n407 = Bundle("Begin (V)"="Begin (V)", w715, w721) -> (→"MCL Scan":cluster{"Begin (V)":dbl, dbl, dbl[]})  [unwired: 1 out]
                n408 = Bundle("Begin (V)"="Begin (V)", w715, w714) -> (→"MCL Scan 2":cluster{"Begin (V)":dbl, dbl, dbl[]})  [unwired: 1 out]
              }
            }
          }
        }
        n409 = local read "Stop All"() -> (w659:bool)
        n410 = node-c288() -> ()  [unwired: 2 out]
      }
      n411 = node-c288(w656) -> ()  [unwired: 1 out]
    }
    frame Disabled {
    }
  }
  n412 = node-c288(2 ("Processor")) -> (w35:T25)  [unwired: 3 in]
  n413 = node-c288() -> (w89:T25)  [unwired: 4 in]
  n414 = timed-loop "Control parameters (event loop)" {
    tunnel: w44 -> [w755]
    shift-right: [w754] -> _
    shift-left: errorcluster {"status"=FALSE, "code"=0, "source"=""} ("error out") -> [w753]
    tunnel: [w752] -> w57
    timing: w35 -> [_]
    timing-out: [_] -> w34
    stop <- w752 stop-if-true
    n415 = node-c288() -> ()  [unwired: 1 in, 1 out]
    n416 = event shown="[54] \"Simulate stepping\": Value Change" {
      selector: _ -> [_ _ _ _ _ _ _ _ _ _ _ _ _ _ _ _ _ _ _ _ _ _ _ _ _ _ _ _ _ _ _ _ _ _ _ _ _ _ _ _ _ _ _ _ _ _ _ _ _ _ _ _ _ _ _ _ _ _ _ _ _]
      dyn-events: _ -> [_ _ _ _ _ _ _ _ _ _ _ _ _ _ _ _ _ _ _ _ _ _ _ _ _ _ _ _ _ _ _ _ _ _ _ _ _ _ _ _ _ _ _ _ _ _ _ _ _ _ _ _ _ _ _ _ _ _ _ _ _]
      timeout: _ -> [_ _ _ _ _ _ _ _ _ _ _ _ _ _ _ _ _ _ _ _ _ _ _ _ _ _ _ _ _ _ _ _ _ _ _ _ _ _ _ _ _ _ _ _ _ _ _ _ _ _ _ _ _ _ _ _ _ _ _ _ _]
      tunnel: w755 -> [w793 _ _ _ w830 _ w848 w854 _ w928 _ _ _ w971 _ _ w1014 w1020 w1025 w1031 w1067 w1085 w1092 w1110 w1121 w1132 w1143 w1154 w1165 w1183 w1189 w1283 _ w1292 w1330 _ w1390 w1394 w1405 w1409 w1413 _ w1421 _ _ _ _ _ w1557 _ w1574 w1589 w1615 w1618 w1619 w1679 _ w1696 w1730 _ _]
      tunnel: [w792 _ _ _ w820 _ _ w853 _ w891 _ w936 _ w950 _ _ w1013 w1016 w1022 w1028 w1066 w1083 w1091 w1104 w1115 w1126 w1137 w1148 w1159 w1181 w1188 w1281 _ w1290 w1328 _ w1388 w1392 w1395 w1407 w1411 _ w1419 _ _ _ _ _ w1555 _ _ _ _ _ _ _ _ _ _ _ _] -> w754
      tunnel: w753 -> [w791 _ _ _ w829 _ _ w852 _ w923 _ w936 _ w970 _ _ w1012 w1015 w1021 w1027 w1065 w1084 w1090 w1109 w1120 w1131 w1142 w1153 w1164 w1182 w1187 w1282 _ w1291 w1329 _ w1389 w1393 w1404 w1408 w1412 _ w1420 _ _ _ _ _ w1556 _ w1573 w1588 w1614 w1617 w1620 w1678 _ w1695 _ _ _]
      tunnel: [_ _ _ _ _ _ _ _ _ _ _ w935 _ _ _ _ _ _ _ _ _ _ _ _ _ _ _ _ _ _ _ _ _ _ _ _ _ _ _ _ _ _ _ _ _ _ _ _ _ _ _ _ _ _ _ _ _ _ _ _ _] -> w752
      tunnel: [_ _ _ _ _ _ _ _ "Round T1 X" _ _ _ _ _ _ _ _ _ _ _ _ _ _ _ _ _ _ _ _ _ _ _ _ _ _ _ _ _ _ _ _ _ _ _ _ _ _ _ _ _ _ _ _ _ _ _ _ _ _ _ _] -> _
      tunnel: [_ _ _ "Adjust Scale\nto Mean" _ _ _ _ _ _ _ _ _ _ _ _ _ _ _ _ _ _ _ _ _ _ _ _ _ _ _ _ _ _ _ _ _ _ _ _ _ _ _ _ _ _ _ _ _ _ _ _ _ _ _ "Set SP to Reading" _ _ _ _ _] -> _
      tunnel: [_ _ _ _ _ _ _ _ _ _ "Round T2 X" _ "Delayed Interlace Start" _ _ _ _ _ _ _ _ _ _ _ _ _ _ _ _ _ _ _ _ _ _ _ _ _ _ _ _ _ _ _ _ _ _ _ _ _ _ _ _ _ _ _ _ _ _ _ _] -> _
      event "AI Count (ticks)", "Sets to FIFO (Traps)", "Save ave N", "FPGA Ave.", "# Samples/channel", "N sets to save": Value Change {
        # "So that if 'Save ave N' is updated, the AOD scanning code updates too."
        n417 = event-data() -> ()  [unwired: 6 out]
        n418 = local read "AI Count (ticks)"() -> (w773:u32)
        n419 = Boolean To (0,1)(Boolean="Sets to FIFO (Traps)") -> (0, 1=w783:cluster{"Set 1":i16, "Set 2":i16, "Set 3":i16})
        n420 = xnode "Read/Write Control"("FPGA VI Reference In"=w793, "error in"=w791, "ai count"=w773, "AI1 Sets to FIFO"="Sets to FIFO (Traps)", "N of AI1 Int Acq Sets"="N Acq Sets (Traps + Fl.)") -> ("error out"=w792:errorcluster)  [unwired: 1 out]
        n421 = Cluster To Array(cluster=w783) -> (array=w782:i16[])
        n422 = To Unsigned Long Integer(number=w782) -> (unsigned 32bit integer=w762:u32[])
        n423 = local read "Scan steps (AOD)"() -> (w784:u64)
        n424 = Multiply(x=w773, y="N Acq Sets (Traps + Fl.)") -> (x*y=w771:u32)
        n425 = Divide(x=40000000.0, y=w773) -> (x/y=w765:dbl)
        "AI rate (Hz)" <- w765
        "Ave. Rate (Hz)" <- w765
        n426 = Add Array Elements(numeric array=w762) -> (sum=w774:u32)
        "Trap Sets" <- w774
        n427 = Reciprocal(x=w765) -> (1/x=→"Ave. Period (s)":dbl)
        n428 = property on="Scan steps (AOD)" class="DigNum (strict)"("Val(Sgnl)"=w784) -> ()  [unwired: 2 in, 2 out]
        n429 = Divide(x=w765, y="N Acq Sets (Traps + Fl.)") -> (x/y=w788:dbl)
        "Data Rate (Hz)" <- w788
        n430 = Reciprocal(x=w788) -> (1/x=→"Data Period (s)":dbl)
        n431 = local read "Save ave N"() -> (w787:dbl)
        n432 = Divide(x=w788, y=w787) -> (x/y=w786:dbl)
        "Save Data Rate (Hz)" <- w786
        n433 = Reciprocal(x=w786) -> (1/x=→"Save Data Period (s)":dbl)
        n434 = Multiply(x=w771, y="# Samples/trap") -> (x*y=w769:u32)
        "Counts/DMA" <- w769
        n435 = property on="Trap Disp. Downsample" class="DigNum (strict)"("Maximum"="# Samples/trap") -> ()  [unwired: 2 in, 2 out]
        n436 = Multiply(x=w774, y="# Samples/trap") -> (x*y=w763:u32)
        "# Samples/channel" <- w763
        n437 = Multiply(x=w763, y=u32 8) -> (x*y=→"Trap AI Elements/DMA read":u32)
        n438 = local read "APD Int. Count"() -> (w770:u32)
        n439 = Multiply(x=w763, y=u32 3) -> (x*y=→"Trap Pos Elements/DMA read":u32)
        n440 = Divide(x=w769, y=w770) -> (x/y=w760:dbl)
        "APD Samples/FIFO Acq." <- w760
        n441 = Divide(x=w769, y=40000000.0) -> (x/y=w767:dbl)
        "DMA Update Period (s)" <- w767
        n442 = Multiply(x=2.0, y=w760) -> (x*y=→"APD Elements/DMA read":dbl)
        n443 = property on="APD Disp. Downsample" class="DigNum (strict)"("Maximum"=w760) -> ()  [unwired: 2 in, 2 out]
        n444 = local read "N sets to save"() -> (w780:u32)
        n445 = Multiply(x=w767, y=w780) -> (x*y=→"Total Time (s)":dbl)
        "FPGA Averaging" <- FALSE ("FPGA Averaging")
      }
      event "Rescale on Mean": Value Change {
        n446 = event-data() -> ()  [unwired: 7 out]
        n447 = And(x=FALSE, y="Rescale on Mean") -> (x .and. y?=w795:bool)
        n448 = local write "Rescale on Mean"(w795) -> ()
        n449 = local read "Bead Mean (nm)"() -> (w800:dbl)
        n450 = Add(x="Amplitude (nm)", y=w800) -> (x+y=w798:dbl)
        n451 = Subtract(x=w800, y="Amplitude (nm)") -> (x-y=w797:dbl)
        n452 = property on="Bead Separation" class="WFChart (strict)"("YScale.Minimum"=w797) -> ()  [unwired: 2 in, 2 out]
        n453 = property on="Bead Separation" class="WFChart (strict)"("YScale.Maximum"=w798) -> ()  [unwired: 2 in, 2 out]
      }
      event "Detector Type": Value Change {
        n454 = event-data() -> ()  [unwired: 7 out]
        n455 = local read "AI labels"() -> (w801:string[])
        n456 = property on="High Res. Display" class="Ring (strict)"("Strings []"=w801) -> ()  [unwired: 2 in, 2 out]
        n457 = Build Array (concatenate)(w801, "none") -> (w802:string[])
        n458 = property on="FFT 1 Choice 1" class="Ring (strict)"("Strings []"=w802) -> ()  [unwired: 2 in, 2 out]
        n459 = property on="FFT 1 Choice 2" class="Ring (strict)"("Strings []"=w802) -> ()  [unwired: 2 in, 2 out]
        n460 = property on="FFT 2 Choice 1" class="Ring (strict)"("Strings []"=w802) -> ()  [unwired: 2 in, 2 out]
        n461 = property on="FFT 2 Choice 2" class="Ring (strict)"("Strings []"=w802) -> ()  [unwired: 2 in, 2 out]
        n462 = Bundle("APD 1", "APD 2") -> (w805:cluster{string, string})  [unwired: 1 out]
        n463 = Cluster To Array(cluster=w805) -> (array=w803:string[])
        n464 = Build Array (concatenate)(w803, w802) -> (w807:string[])
        n465 = Array Size(array=w807) -> (size(s)=w808:i32)
        n466 = property on="Signals to Plot" class="LstBox (strict)"("Item Names"=w807) -> ()  [unwired: 2 in, 2 out]
        n467 = property on="Signals to Plot" class="LstBox (strict)"("Number of Rows"=w808) -> ()  [unwired: 2 in, 2 out]
        n468 = property on="All Signals" class="WFChart (strict)"("LegNumRows"=w808) -> ()  [unwired: 2 in, 2 out]
      }
      event "Adjust Scale\nto Mean": Value Change {
        n469 = event-data() -> ()  [unwired: 7 out]
        n470 = local read "APD 1 Rate (Hz)"() -> (w817:dbl)
        n471 = Multiply(x=1000.0, y="Above (kHz)") -> (x*y=w815:dbl)
        n472 = Multiply(x=1000.0, y="Below (kHz)") -> (x*y=w813:dbl)
        n473 = Add(x=w815, y=w817) -> (x+y=w810:dbl)
        n474 = Subtract(x=w817, y=w813) -> (x-y=w811:dbl)
        n475 = property on="APD Chart" class="WFChart (strict)"("YScale.Minimum"=w811) -> ()  [unwired: 2 in, 2 out]
        n476 = property on="APD Chart" class="WFChart (strict)"("YScale.Maximum"=w810) -> ()  [unwired: 2 in, 2 out]
      }
      event "Phase adj. (AI1)", "+ phase (AI1)", "- phase (AI1)": Value Change {
        n477 = event-data() -> ()  [unwired: 7 out]
        n478 = Negate(x="Phase adj. (AI1)") -> (-x=w827:i16)
        n479 = Select(t=w827, s="- phase (AI1)", f="Phase adj. (AI1)") -> (s? t:f=w826:i16)
